vi "CustomPID_v4.1.vi"(0 "PID Tuning Parameters":T1={"Kp"=0.1, "Ki"=0.1, "Kd"=0.1, "N-Diff"=10, "N-Int"=20, "Int Error Window"=0.5, "Max Ouput"=1.0, "Min Output"=-1.0, "Square Derivative"=FALSE, "N-Prop"=1} {"N-Prop" min=1; "Int Error Window" min=0.0; "N-Int" min=2; "N-Diff" min=2; "Kd" min=0.0; "Ki" min=0.0; "Kp" min=0.0}, 1 "Goal":dbl(slide) scale=-1.0..1.0, 2 "Process Variable":dbl(slide) scale=-1.0..1.0, 3 "Custom Error Calculation":dbl(slide) scale=-1.0..1.0, 7 "Reset on Goal Change ?":bool, 9 "Use Custom Error Calculation ?":bool, 12 "Reinit":bool) -> (4 "Command":dbl format="%_4g", 6 "Is Reset":bool, 8 "Current Error":dbl format="%_4g", 15 "Controller Summary":T2(graph))   [LabVIEW 2023]
doc: "A custom PID implimentation with several modifications for working with common FRC applications. The custom error calculation should be used when working with a wrapping goal (e.g., maintaining a rotational position). The integral error window can be used to prevent integrator windup. Squaring the derivative can increase the sensivity to rapid changes in the error. An exponential decay can be applied to the proportional calculation to weight more recent errors more heavily.\n\nA good mechanical analogy for a PID algorithm is a spring-mass system with a viscous damper \n(https://ccrma.stanford.edu/CCRMA/Courses/150/img35.gif). The proportional term is the \"spring,\" it has the strongest influence when the robot system is furthest from its goal. The derivative term is the damping coefficient, it's what allows the system to stop oscillating and reach it's goal. The integral term mostly comes into play if the robot has been been trying to move for a lengthy amount of time but still isn't able to reach it's goal (this is referred to as steady-state error).\n\nRecommended Tuning Procedure:\n\n1) You may want to restrict the Max and Min Output parameters more than [-1, 1] during initial tuning to avoid damaging the system.\n2) Carefully increase the Kp term from 0.0001 until the system starts moving.\n3) If the system is going the wrong direction, you may need to negate the Command.\n4) Continue inceasing Kp until the system oscillates about the Goal.\n5) Carefully increase Kd from 0.0001 until the system's response is sufficiently damped (i.e. until the oscillation is mitigated).\n6) Carefully increase Ki from 0.0001 to reduce the steady-state error (SSE) (if any).\n7) Adjust N-Diff if necessary (minimum of 2). Increasing N-Diff will reduce the effects of sensor (Process Variable) noise on the \nderivative term but will increase the lag on that component. You may also want to add a filter to Process Variable data.\n8) Adjust N-Int if necessary (minimum of 2). Increasing N-Int may help the system overcome SSE but may also increase integrator wind-up. It will also increase the lag for that component.\n9) Another way to reduce integrator wind-up is to set the Integral Error Window. The Intergral term will only be used if the magnitude of the error is less than the specified window.\n10) You may need to adjust Kp, Ki, and Kd after adjusting N-Diff and N-Int."
uses:
  <vilib>/Analysis/6fits.llb/Curve Fitting Criteria.ctl
  <vilib>/Analysis/4window.llb/Exponential Window (DBL).vi
  <vilib>/Analysis/NI_AALPro.lvlib
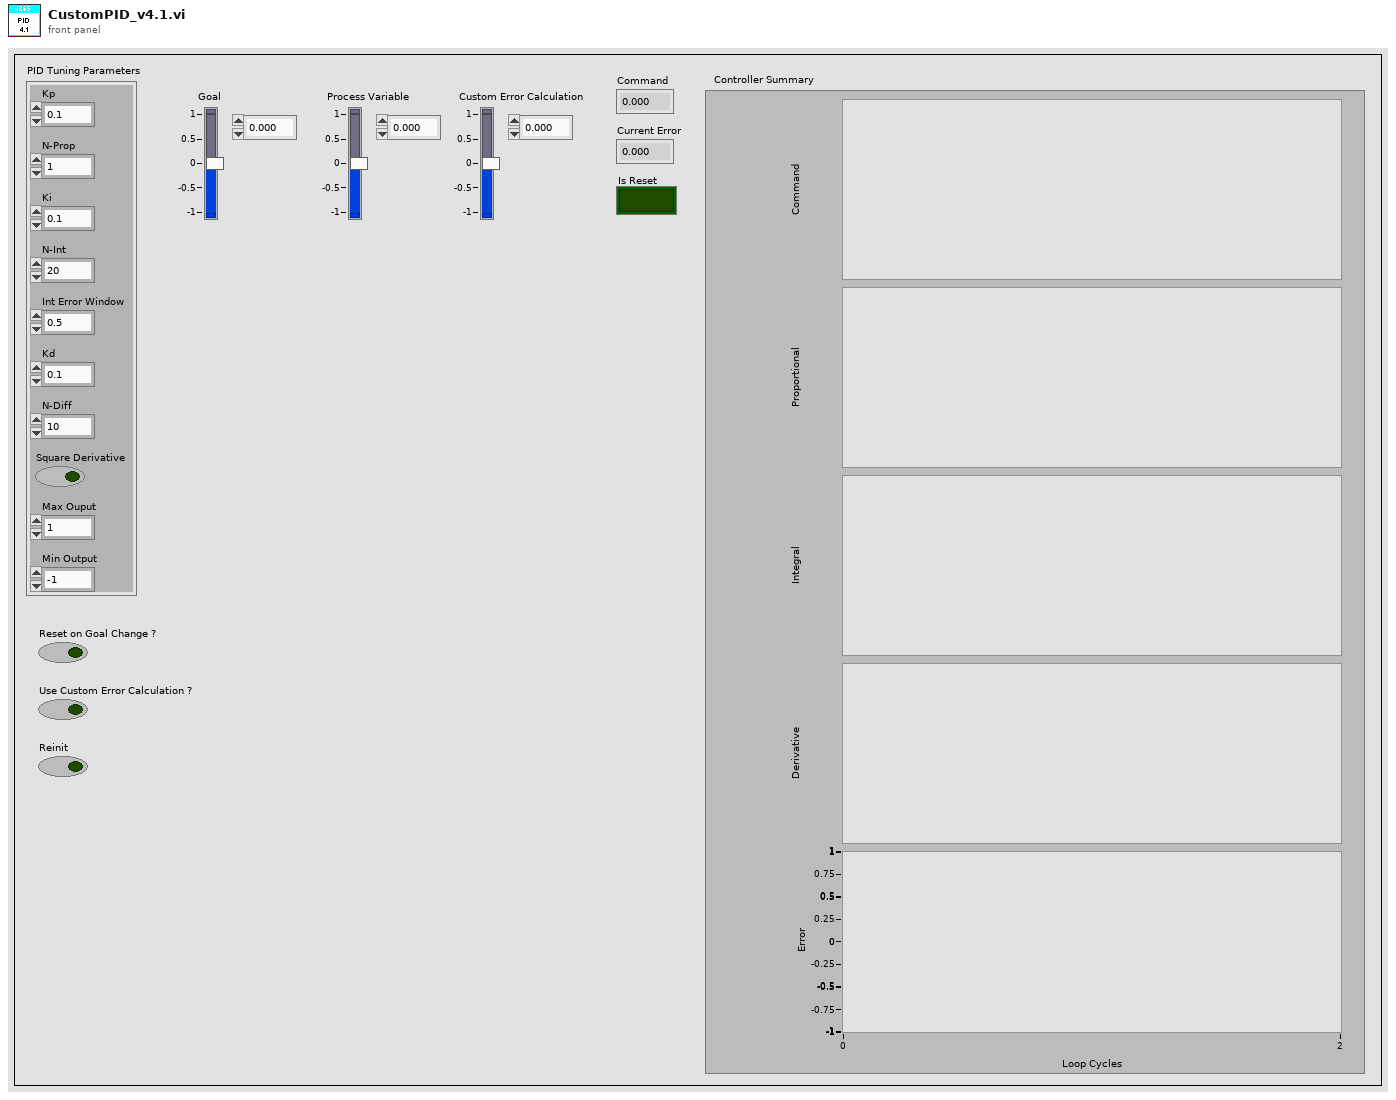
[diagram p1: front panel]
types:
  T1 = cluster{"Kp":dbl, "Ki":dbl, "Kd":dbl, "N-Diff":i32, "N-Int":i32, "Int Error Window":dbl, "Max Ouput":dbl, "Min Output":dbl, "Square Derivative":bool, "N-Prop":i32}
  T2 = cluster{"Command":dbl, "Proportional":dbl, "Integral":dbl, "Derivative":dbl, "Goal":dbl}
  T3 = cluster{"Command":dbl, "Proportional":dbl, "Integral":dbl, "Derivative":dbl, "Error":dbl}
  T4 = typedef "NI_AALPro.lvlib/Curve Fitting Criteria.ctl" = u16
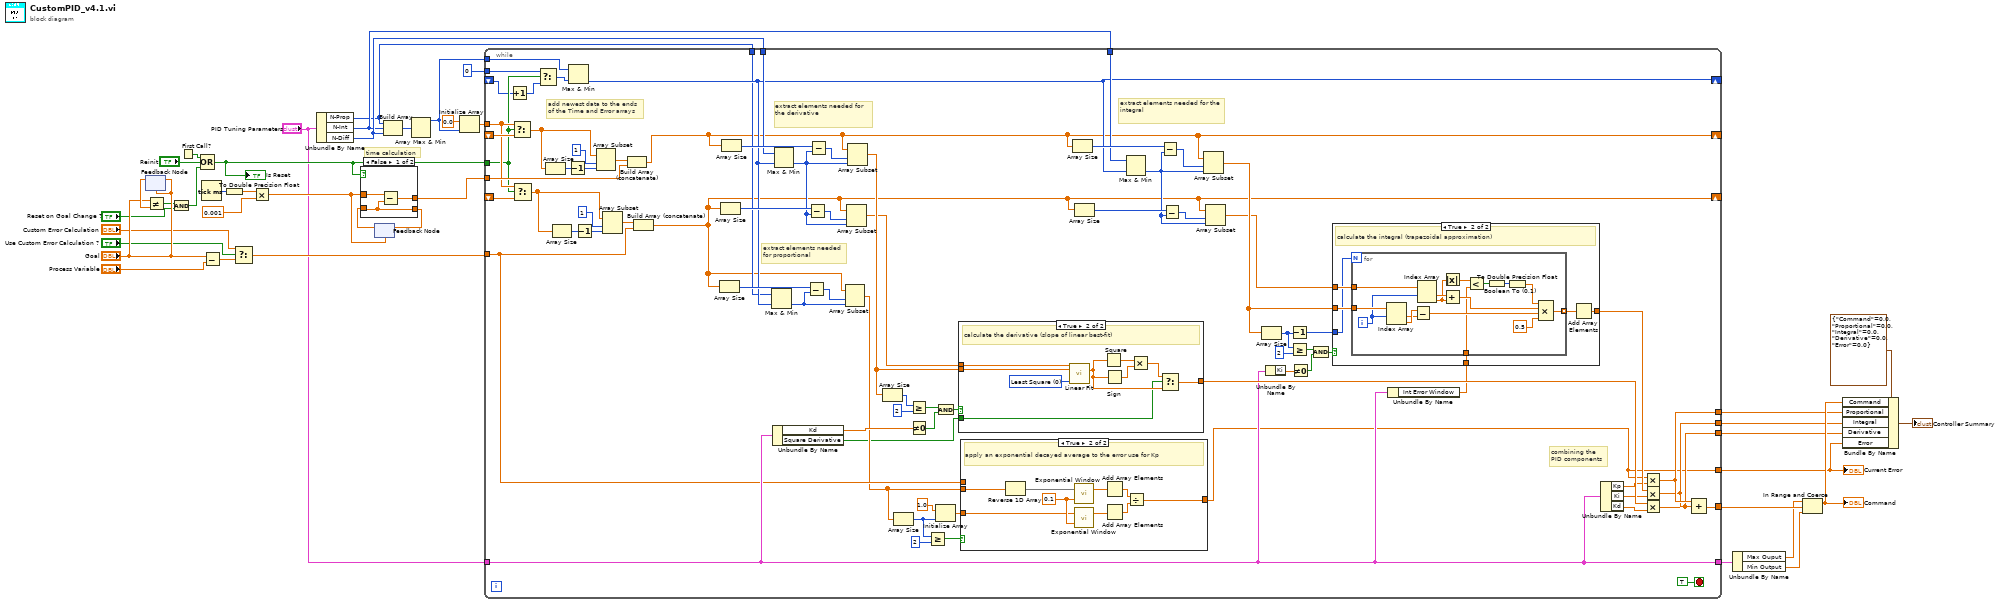
[diagram p0: block diagram]
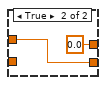
[diagram p2: hidden frame]
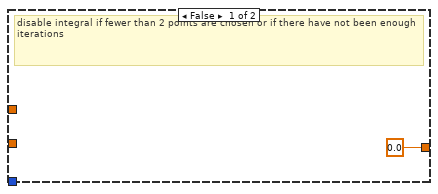
[diagram p4: hidden frame]
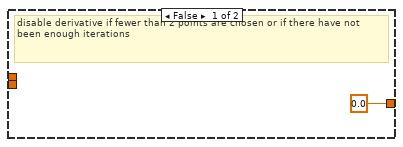
[diagram p5: hidden frame]
diagram:
  # "time calculation"
  n1 = feedback #1("Goal") -> (w35:dbl)
  n2 = feedback-in #1("Goal") -> ()
  n3 = Not Equal?(x="Goal", y=w35) -> (x != y?=w18:bool)
  n4 = And(x=w18, y="Reset on Goal Change ?") -> (x .and. y?=w28:bool)
  n5 = First Call?() -> (First Call?: T/F=w39:bool)
  n6 = Compound Arithmetic op=OR(w39, "Reinit", w28) -> (w29:bool)
  "Is Reset" <- w29
  n7 = Tick Count (ms)() -> (millisecond timer value=w34:u32)
  n8 = Subtract(x="Goal", y="Process Variable") -> (x-y=w16:dbl)
  n9 = To Double Precision Float(number=w34) -> (double precision float=w33:dbl)
  n10 = Select(t="Custom Error Calculation", s="Use Custom Error Calculation ?", f=w16) -> (s? t:f=w15:dbl)
  n11 = Multiply(x=w33, y=0.001) -> (x*y=w27:dbl)
  n12 = Unbundle By Name("PID Tuning Parameters") -> ("N-Prop"=w2:i32, "N-Int"=w5:i32, "N-Diff"=w6:i32)
  n13 = feedback #2(w27) -> (w30:dbl)
  n14 = case shown="False" w29 {
    tunnel: w27 -> [w43 w45]
    tunnel: [w41 w45] -> w31
    tunnel: [w42 0.0] -> w21
    tunnel: w30 -> [w41 _]
    frame False {
      n15 = Subtract(x=w43, y=w41) -> (x-y=w42:dbl)
    }
    frame True {
    }
  }
  n16 = feedback-in #2(w31) -> ()
  n17 = Build Array(w2, w5, w6) -> (w4:i32[])
  n18 = Array Max & Min(array=w4) -> (max value=w3:i32)  [unwired: 3 out]
  n19 = Initialize Array(0.0 ("element"), w3) -> (w37:dbl[])
  n20 = while {
    tunnel: [w121] -> w40
    tunnel: w15 -> [w59]
    shift-right: [w49] -> _
    shift-left: _ -> [w98]
    tunnel: w21 -> [w116]
    shift-right: [w48] -> _
    shift-left: _ -> [w95]
    tunnel: w29 -> [w87]
    tunnel: w37 -> [w96]
    tunnel: [w58] -> w12
    tunnel: [w91] -> w25
    tunnel: [w90] -> w24
    tunnel: [w89] -> w23
    tunnel: 0 -> [w88]
    shift-right: [w51] -> _
    shift-left: _ -> [w85]
    tunnel: w3 -> [w82]
    tunnel: w5 -> [w72]
    tunnel: w6 -> [w71]
    tunnel: "PID Tuning Parameters" -> [w64]
    tunnel: [w64] -> w9
    tunnel: w2 -> [w50]
    stop <- TRUE stop-if-true
    # "extract elements needed\nfor proportional"
    # "combining the\nPID components"
    # "add newest data to the ends\nof the Time and Error arrays"
    # "extract elements needed for the integral"
    # "extract elements needed for the derivative"
    n21 = Increment(x=w85) -> (x+1=w86:i32)
    n22 = Select(t=w96, s=w87, f=w98) -> (s? t:f=w97:dbl[])
    n23 = Select(t=w96, s=w87, f=w95) -> (s? t:f=w94:dbl[])
    n24 = Select(t=w88, s=w87, f=w86) -> (s? t:f=w83:i32)
    n25 = Array Size(array=w97) -> (size(s)=w119:i32)
    n26 = Array Size(array=w94) -> (size(s)=w114:i32)
    n27 = Decrement(x=w119) -> (x-1=w118:i32)
    n28 = Max & Min(x=w82, y=w83) -> (min(x,y)=w51:i32)  [unwired: 1 out]
    n29 = Decrement(x=w114) -> (x-1=w113:i32)
    n30 = Array Subset(array=w97, index=1, length=w118) -> (w117:dbl[])
    n31 = Array Subset(array=w94, index=1, length=w113) -> (w112:dbl[])
    n32 = Build Array (concatenate)(w117, w116) -> (w49:dbl[])
    n33 = Build Array (concatenate)(w112, w59) -> (w48:dbl[])
    n34 = Array Size(array=w48) -> (size(s)=w54:i32)
    n35 = Array Size(array=w48) -> (size(s)=w108:i32)
    n36 = Array Size(array=w49) -> (size(s)=w111:i32)
    n37 = Max & Min(x=w50, y=w51) -> (min(x,y)=w52:i32)  [unwired: 1 out]
    n38 = Unbundle By Name(w64) -> ("Kd"=w70:dbl, "Square Derivative"=w46:bool)
    n39 = Max & Min(x=w71, y=w51) -> (min(x,y)=w84:i32)  [unwired: 1 out]
    n40 = Subtract(x=w54, y=w52) -> (x-y=w53:i32)
    n41 = Subtract(x=w108, y=w84) -> (x-y=w109:i32)
    n42 = Subtract(x=w111, y=w84) -> (x-y=w110:i32)
    n43 = Array Subset(array=w48, index=w53, length=w52) -> (w47:dbl[])
    n44 = Array Subset(array=w48, index=w109, length=w84) -> (w61:dbl[])
    n45 = Array Subset(array=w49, index=w110, length=w84) -> (w107:dbl[])
    n46 = Array Size(array=w107) -> (size(s)=w62:i32)
    n47 = Array Size(array=w47) -> (size(s)=w56:i32)
    n48 = Greater Or Equal?(x=w62, y=2) -> (x >= y?=w81:bool)
    n49 = Not Equal To 0?(x=w70) -> (x != 0?=w79:bool)
    n50 = Greater Or Equal?(x=w56, y=2) -> (x >= y?=w55:bool)
    n51 = Initialize Array(1.0 ("element"), w56) -> (w60:dbl[])
    n52 = Compound Arithmetic op=AND(w81, w79) -> (w80:bool)
    n53 = case shown="True" w80 {
      tunnel: w61 -> [_ w163]
      tunnel: w107 -> [_ w164]
      tunnel: [0.0 w159] -> w92
      tunnel: w46 -> [_ w157]
      frame False {
        # "disable derivative if fewer than 2 points are chosen or if there have not been enough iterations"
      }
      frame True {
        w165 = T4 0 items=["Least Square", "Least Absolute Residual", "Bisquare"] ("method")
        # "calculate the derivative (slope of linear best-fit)"
        n54 = call <vilib>:"Linear Fit.vi"("Y"=w163, "X"=w164, "method"=w165) -> ("slope"=w158:dbl)  [unwired: 8 in, 4 out]
        n55 = Square(x=w158) -> (x^2=w161:dbl)
        n56 = Sign(1:w158) -> (0:w162:dbl)
        n57 = Multiply(x=w161, y=w162) -> (x*y=w160:dbl)
        n58 = Select(t=w160, s=w157, f=w158) -> (s? t:f=w159:dbl)
      }
    }
    n59 = case shown="True" w55 {
      tunnel: w47 -> [_ w126]
      tunnel: w60 -> [_ w125]
      tunnel: w59 -> [w123 _]
      tunnel: [w123 w124] -> w58
      frame False {
        # "disable error averaging if fewer than 2 points are chosen or if there have not been enough iterations"
      }
      frame True {
        w131 = 0.1 ("final value")
        # "apply an exponential decayed average to the error use for Kp"
        n60 = Reverse 1D Array(array=w126) -> (reversed array=w127:dbl[])
        n61 = call-poly <vilib>:"Exponential Window.vi"("final value"=w131, "X"=w127) -> ("Windowed X"=w132:dbl[])  [unwired: 1 out]
        n62 = call-poly <vilib>:"Exponential Window.vi"("final value"=w131, "X"=w125) -> ("Windowed X"=w130:dbl[])  [unwired: 1 out]
        n63 = Add Array Elements(numeric array=w132) -> (sum=w129:dbl)
        n64 = Add Array Elements(numeric array=w130) -> (sum=w128:dbl)
        n65 = Divide(x=w129, y=w128) -> (x/y=w124:dbl)
      }
    }
    n66 = Array Size(array=w49) -> (size(s)=w105:i32)
    n67 = Array Size(array=w48) -> (size(s)=w103:i32)
    n68 = Max & Min(x=w72, y=w51) -> (min(x,y)=w78:i32)  [unwired: 1 out]
    n69 = Subtract(x=w105, y=w78) -> (x-y=w104:i32)
    n70 = Subtract(x=w103, y=w78) -> (x-y=w102:i32)
    n71 = Array Subset(array=w49, index=w104, length=w78) -> (w99:dbl[])
    n72 = Array Subset(array=w48, index=w102, length=w78) -> (w93:dbl[])
    n73 = Array Size(array=w99) -> (size(s)=w77:i32)
    n74 = Unbundle By Name(w64) -> ("Ki"=w69:dbl)
    n75 = Decrement(x=w77) -> (x-1=w76:i32)
    n76 = Greater Or Equal?(x=w77, y=2) -> (x >= y?=w75:bool)
    n77 = Not Equal To 0?(x=w69) -> (x != 0?=w73:bool)
    n78 = Compound Arithmetic op=AND(w75, w73) -> (w74:bool)
    n79 = Unbundle By Name(w64) -> ("Int Error Window"=w68:dbl)
    n80 = case shown="True" w74 {
      tunnel: [0.0 w134] -> w100
      tunnel: w99 -> [_ w139]
      tunnel: w93 -> [_ w138]
      tunnel: w68 -> [_ w137]
      tunnel: w76 -> [_ w136]
      frame False {
        # "disable integral if fewer than 2 points are chosen or if there have not been enough iterations"
      }
      frame True {
        # "calculate the integral (trapezoidal approximation)"
        n81 = for {
          N: w136 -> [_]
          tunnel: w139 -> [w155]
          tunnel: w138 -> [w149]
          tunnel: w137 -> [w142]
          tunnel: [w141] -> w135 mode=indexing
          i -> [w150]
          n82 = Index Array(array=w155, index #1=w150) -> (element #1=w153:dbl, element #2=w154:dbl)  [unwired: 1 in]
          n83 = Subtract(x=w154, y=w153) -> (x-y=w152:dbl)
          n84 = Index Array(array=w149, index #1=w150) -> (element #1=w147:dbl, element #2=w140:dbl)  [unwired: 1 in]
          n85 = Absolute Value(x=w140) -> (abs(x)=w146:dbl)
          n86 = Add(x=w147, y=w140) -> (x+y=w148:dbl)
          n87 = Less?(x=w146, y=w142) -> (x < y?=w145:bool)
          n88 = Boolean To (0,1)(Boolean=w145) -> (0, 1=w144:i16)
          n89 = To Double Precision Float(number=w144) -> (double precision float=w143:dbl)
          n90 = Compound Arithmetic op=MULTIPLY(w143, w148, w152, 0.5 ("value")) -> (w141:dbl)
        }
        n91 = Add Array Elements(numeric array=w135) -> (sum=w134:dbl)
      }
    }
    n92 = Unbundle By Name(w64) -> ("Kp"=w67:dbl, "Ki"=w66:dbl, "Kd"=w65:dbl)
    n93 = Multiply(x=w58, y=w67) -> (x*y=w91:dbl)
    n94 = Multiply(x=w100, y=w66) -> (x*y=w90:dbl)
    n95 = Multiply(x=w92, y=w65) -> (x*y=w89:dbl)
    n96 = Compound Arithmetic op=ADD(w91, w90, w89) -> (w121:dbl)
  }
  "Current Error" <- w12
  n97 = Unbundle By Name(w9) -> ("Max Ouput"=w8:dbl, "Min Output"=w7:dbl)
  n98 = In Range and Coerce(upper limit=w8, x=w40, lower limit=w7) -> (coerced(x)=w26:dbl)  [unwired: 1 out]
  "Command" <- w26
  n99 = Bundle By Name(cluster=T3 {"Command"=0.0, "Proportional"=0.0, "Integral"=0.0, "Derivative"=0.0, "Error"=0.0} ("input cluster"), "Command"=w26, "Proportional"=w25, "Integral"=w24, "Derivative"=w23, "Error"=w12) -> (→"Controller Summary":T3)
